vi "Close.vi"(8 "error in":errorcluster, 11 "Engine in":refnum<class "Engine.lvclass">) -> (0 "error out":errorcluster)   [LabVIEW 2017, in "Engine.lvclass"]
uses:
  Engine.lvclass
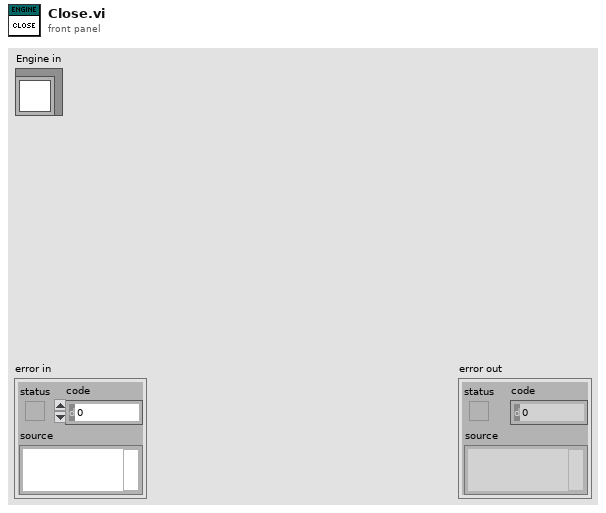
[diagram p1: front panel]
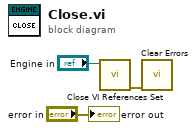
[diagram p0: block diagram]
diagram:
  n1 = call "Close VI References Set.vi"("Engine in"="Engine in") -> ("error out"=w2:errorcluster)  [unwired: 9 in, 1 out]
  n2 = call <vilib>:"Clear Errors.vi"("error in (no error)"=w2) -> ()  [unwired: 5 in, 2 out]
  "error out" <- "error in"
